vi "Core_[HSMS]Not Selected(Passive).vi"(8 "error in (no error)":errorcluster, 11 "HSMS Class in":refnum<class "HSMS Class.lvclass">) -> (0 "error out":errorcluster, 3 "HSMS Class out":refnum<class "HSMS Class.lvclass">)   [LabVIEW 2020, in "SECS Communication.lvlib" / "HSMS Class.lvclass"]
uses:
  HSMS Class.lvclass
  HSMS Class.lvclass/HSMS Class.ctl
  Notifier Type.ctl
  HSMS State.ctl
  Message Packet.ctl
  Message Header.ctl
  PType.ctl
  SType.ctl
  Read T7(Not Selected Timeout).vi
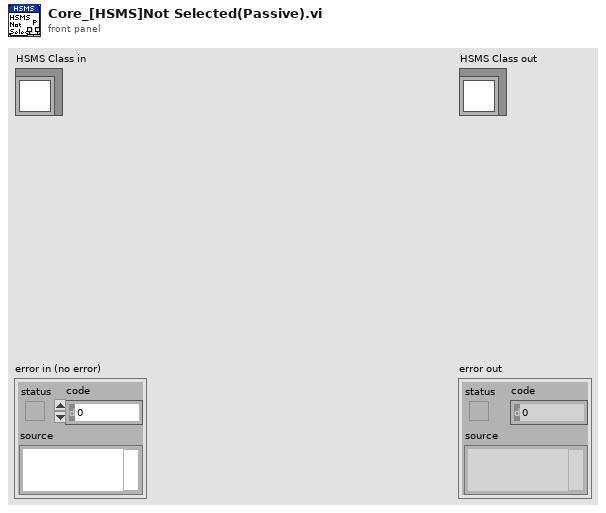
[diagram p1: front panel]
types:
  T1 = typedef "SECS Communication.lvlib/HSMS Class.lvclass/Message Packet.ctl" = cluster{"Message Header Cluster":T2, "Message Header":u8[], "Message Text":u8[]}
  T2 = typedef "SECS Communication.lvlib/HSMS Class.lvclass/Message Header.ctl" = cluster{"Byte 0-1(Session ID)":u16, "W-Bit":bool, "Byte 2":u8, "Byte 3":u8, "Byte 4(PType)":T3, "Byte 5(SType)":T4, "Byte 6-9(System Btyes)":u8[]}
  T3 = typedef "SECS Communication.lvlib/HSMS Class.lvclass/PType.ctl" = enum8{"SECS-II Encoding", "Reserved"}
  T4 = typedef "SECS Communication.lvlib/HSMS Class.lvclass/SType.ctl" = enum8{"Data Message", "Select.req", "Select.rsp", "Deselect.req", "Deselect.rsp", "Linktest.req", "Linktest.rsp", "Reject.req", "Separate.req"}
  T5 = typedef "SECS Communication.lvlib/HSMS Class.lvclass/Notifier Type.ctl" = enum16{"TCPIP Connect", "TCPIP Disconnect", "Receive Message", "Send Message", "T3 Timeout", "T6 Timeout", "T7 Timeout", "Error", "Stop"}
  T6 = typedef "SECS Communication.lvlib/HSMS Class.lvclass/HSMS State.ctl" = enum16{"[TCP/IP]Not Connect", "[HSMS]Not Selected", "[HSMS]Selected", "Stop"}
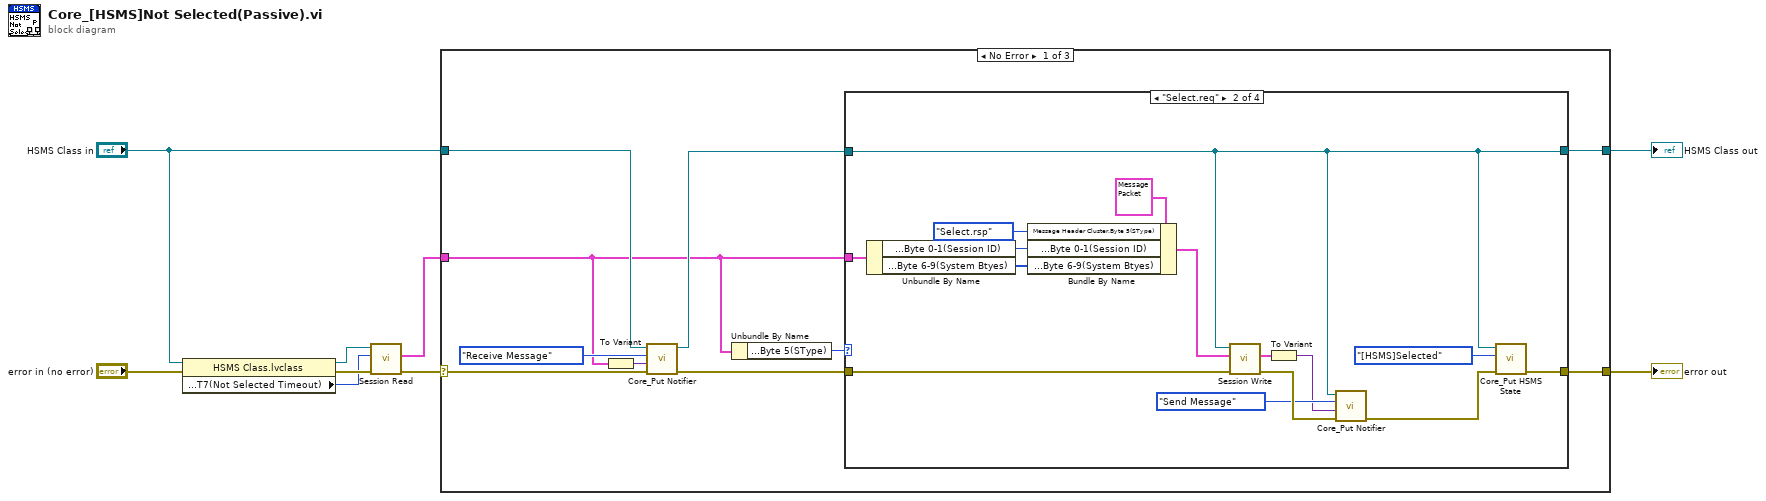
[diagram p0: block diagram]
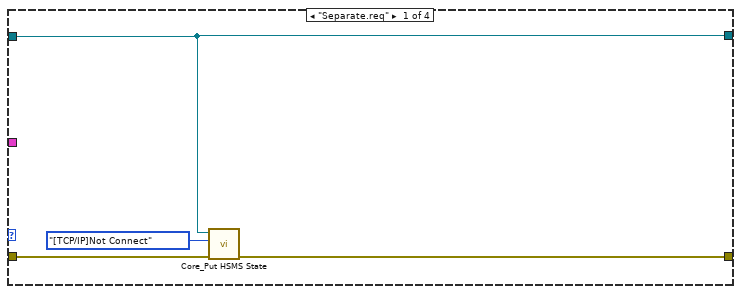
[diagram p2: hidden frame]
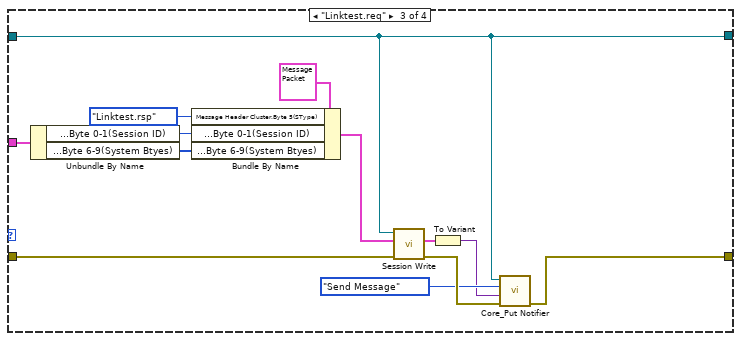
[diagram p3: hidden frame]
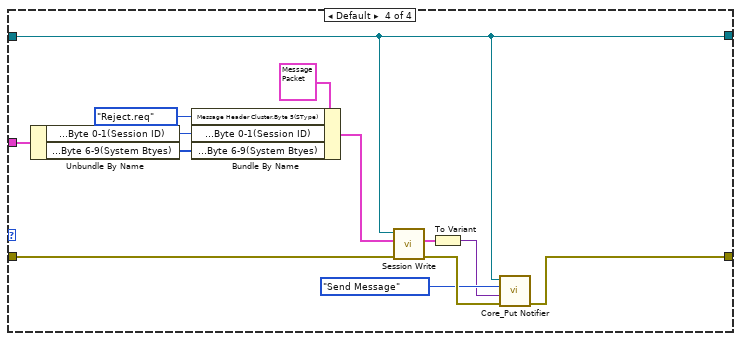
[diagram p4: hidden frame]
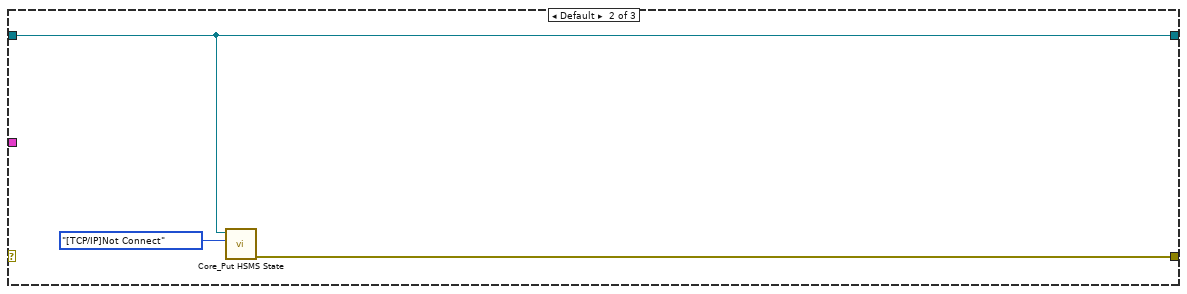
[diagram p5: hidden frame]
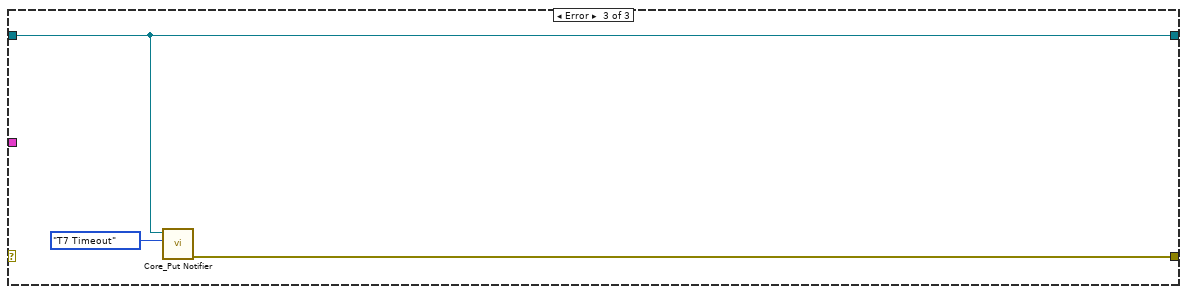
[diagram p6: hidden frame]
diagram:
  n1 = property class="HSMS Class.lvclass"(reference="HSMS Class in", error in="error in (no error)") -> (reference out=w4:refnum<class "HSMS Class.lvclass">, error out=w5:errorcluster, "Public:Property:Setting:T7(Not Selected Timeout)"=w3:i32)
  n2 = call "Session Read.vi"("error in (no error)"=w5, "Timeout"=w3, "HSMS Class in"=w4) -> ("error out"=w2:errorcluster, "Message Packet"=w1:T1)  [unwired: 6 in, 1 out]
  n3 = case shown="No Error" w2 {
    selector: w2 -> [w17 _ _]
    tunnel: w1 -> [w10 _ _]
    tunnel: [w11 w66 w69] -> w8
    tunnel: "HSMS Class in" -> [w18 w65 w68]
    tunnel: [w12 w65 w68] -> w7
    frame No Error {
      n4 = To Variant(anything=w10) -> (Variant=w16:variant)
      n5 = call "Core_Put Notifier.vi"("error in (no error)"=w17, "Data"=w16, "Notifier Type"=Notifier_Type."Receive Message", "HSMS Class in"=w18) -> ("error out"=w15:errorcluster, "HSMS Class out"=w13:refnum<class "HSMS Class.lvclass">)  [unwired: 6 in]
      n6 = Unbundle By Name(w10) -> ("Message Header Cluster.Byte 5(SType)"=w14:T4)
      n7 = case shown="\"Select.req\"" w14 {
        tunnel: w13 -> [w22 w26 w41 w54]
        tunnel: [w22 w26 w41 w54] -> w12
        tunnel: w15 -> [w23 w29 w42 w55]
        tunnel: [w21 w25 w39 w52] -> w11
        tunnel: w10 -> [_ w24 w40 w53]
        frame "Separate.req" {
          n8 = call "Core_Put HSMS State.vi"("error in (no error)"=w23, "HSMS State"=HSMS_State."[TCP/IP]Not Connect", "HSMS Class in"=w22) -> ("error out"=w21:errorcluster)  [unwired: 7 in, 1 out]
        }
        frame "Select.req" {
          n9 = Unbundle By Name(w24) -> ("Message Header Cluster.Byte 0-1(Session ID)"=w37:u16, "Message Header Cluster.Byte 6-9(System Btyes)"=w35:u8[])
          n10 = Bundle By Name(cluster=T1 {"Message Header Cluster"={"Byte 0-1(Session ID)"=0, "W-Bit"=FALSE, "Byte 2"=0, "Byte 3"=0, "Byte 4(PType)"=enum."SECS-II Encoding", "Byte 5(SType)"=enum."Data Message", "Byte 6-9(System Btyes)"=[]}, "Message Header"=[], "Message Text"=[]} ("Message Packet"), "Message Header Cluster.Byte 5(SType)"=SType."Select.rsp" ("Message Header.Byte 5(SType)"), "Message Header Cluster.Byte 0-1(Session ID)"=w37, "Message Header Cluster.Byte 6-9(System Btyes)"=w35) -> (w32:T1)
          n11 = call "Session Write.vi"("error in (no error)"=w29, "Message Packet In"=w32, "HSMS Class in"=w26) -> ("error out"=w34:errorcluster, "Message Packet Out"=w30:T1)  [unwired: 6 in, 1 out]
          n12 = To Variant(anything=w30) -> (Variant=w31:variant)
          n13 = call "Core_Put Notifier.vi"("error in (no error)"=w34, "Data"=w31, "Notifier Type"=Notifier_Type."Send Message", "HSMS Class in"=w26) -> ("error out"=w27:errorcluster)  [unwired: 6 in, 1 out]
          n14 = call "Core_Put HSMS State.vi"("error in (no error)"=w27, "HSMS State"=HSMS_State."[HSMS]Selected", "HSMS Class in"=w26) -> ("error out"=w25:errorcluster)  [unwired: 7 in, 1 out]
        }
        frame "Linktest.req" {
          n15 = Unbundle By Name(w40) -> ("Message Header Cluster.Byte 0-1(Session ID)"=w50:u16, "Message Header Cluster.Byte 6-9(System Btyes)"=w48:u8[])
          n16 = Bundle By Name(cluster=T1 {"Message Header Cluster"={"Byte 0-1(Session ID)"=0, "W-Bit"=FALSE, "Byte 2"=0, "Byte 3"=0, "Byte 4(PType)"=enum."SECS-II Encoding", "Byte 5(SType)"=enum."Data Message", "Byte 6-9(System Btyes)"=[]}, "Message Header"=[], "Message Text"=[]} ("Message Packet"), "Message Header Cluster.Byte 5(SType)"=SType."Linktest.rsp" ("Message Header.Byte 5(SType)"), "Message Header Cluster.Byte 0-1(Session ID)"=w50, "Message Header Cluster.Byte 6-9(System Btyes)"=w48) -> (w45:T1)
          n17 = call "Session Write.vi"("error in (no error)"=w42, "Message Packet In"=w45, "HSMS Class in"=w41) -> ("error out"=w47:errorcluster, "Message Packet Out"=w43:T1)  [unwired: 6 in, 1 out]
          n18 = To Variant(anything=w43) -> (Variant=w44:variant)
          n19 = call "Core_Put Notifier.vi"("error in (no error)"=w47, "Data"=w44, "Notifier Type"=Notifier_Type."Send Message", "HSMS Class in"=w41) -> ("error out"=w39:errorcluster)  [unwired: 6 in, 1 out]
        }
        frame Default {
          n20 = Unbundle By Name(w53) -> ("Message Header Cluster.Byte 0-1(Session ID)"=w63:u16, "Message Header Cluster.Byte 6-9(System Btyes)"=w61:u8[])
          n21 = Bundle By Name(cluster=T1 {"Message Header Cluster"={"Byte 0-1(Session ID)"=0, "W-Bit"=FALSE, "Byte 2"=0, "Byte 3"=0, "Byte 4(PType)"=enum."SECS-II Encoding", "Byte 5(SType)"=enum."Data Message", "Byte 6-9(System Btyes)"=[]}, "Message Header"=[], "Message Text"=[]} ("Message Packet"), "Message Header Cluster.Byte 5(SType)"=SType."Reject.req" ("Message Header.Byte 5(SType)"), "Message Header Cluster.Byte 0-1(Session ID)"=w63, "Message Header Cluster.Byte 6-9(System Btyes)"=w61) -> (w58:T1)
          n22 = call "Session Write.vi"("error in (no error)"=w55, "Message Packet In"=w58, "HSMS Class in"=w54) -> ("error out"=w60:errorcluster, "Message Packet Out"=w56:T1)  [unwired: 6 in, 1 out]
          n23 = To Variant(anything=w56) -> (Variant=w57:variant)
          n24 = call "Core_Put Notifier.vi"("error in (no error)"=w60, "Data"=w57, "Notifier Type"=Notifier_Type."Send Message", "HSMS Class in"=w54) -> ("error out"=w52:errorcluster)  [unwired: 6 in, 1 out]
        }
      }
    }
    frame Default {
      n25 = call "Core_Put HSMS State.vi"("HSMS State"=HSMS_State."[TCP/IP]Not Connect", "HSMS Class in"=w65) -> ("error out"=w66:errorcluster)  [unwired: 8 in, 1 out]
    }
    frame Error {
      n26 = call "Core_Put Notifier.vi"("Notifier Type"=Notifier_Type."T7 Timeout", "HSMS Class in"=w68) -> ("error out"=w69:errorcluster)  [unwired: 8 in, 1 out]
    }
  }
  "error out" <- w8
  "HSMS Class out" <- w7
